vi "Read_File_and_Set_Last_Modified.vi"(5 "file path":path) -> (0 "error out":errorcluster, 1 "string":string, 2 "file path Out":path)   [LabVIEW 2020]
uses:
  Globals/Trav_pos_global.vi
panel:
  out "substring":string
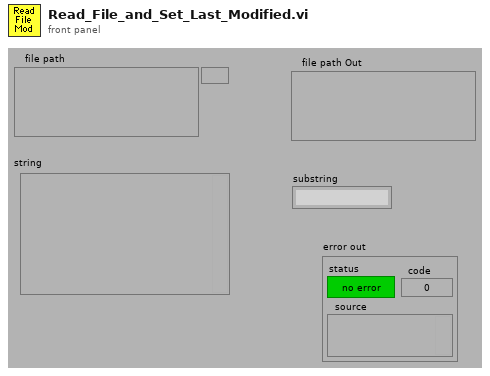
[diagram p1: front panel]
types:
  T1 = enum16{"deny read/write", "deny write-only", "deny none"}
  T2 = enum16{"open", "replace", "create", "open or create", "replace or create", "replace or create with confirmation"}
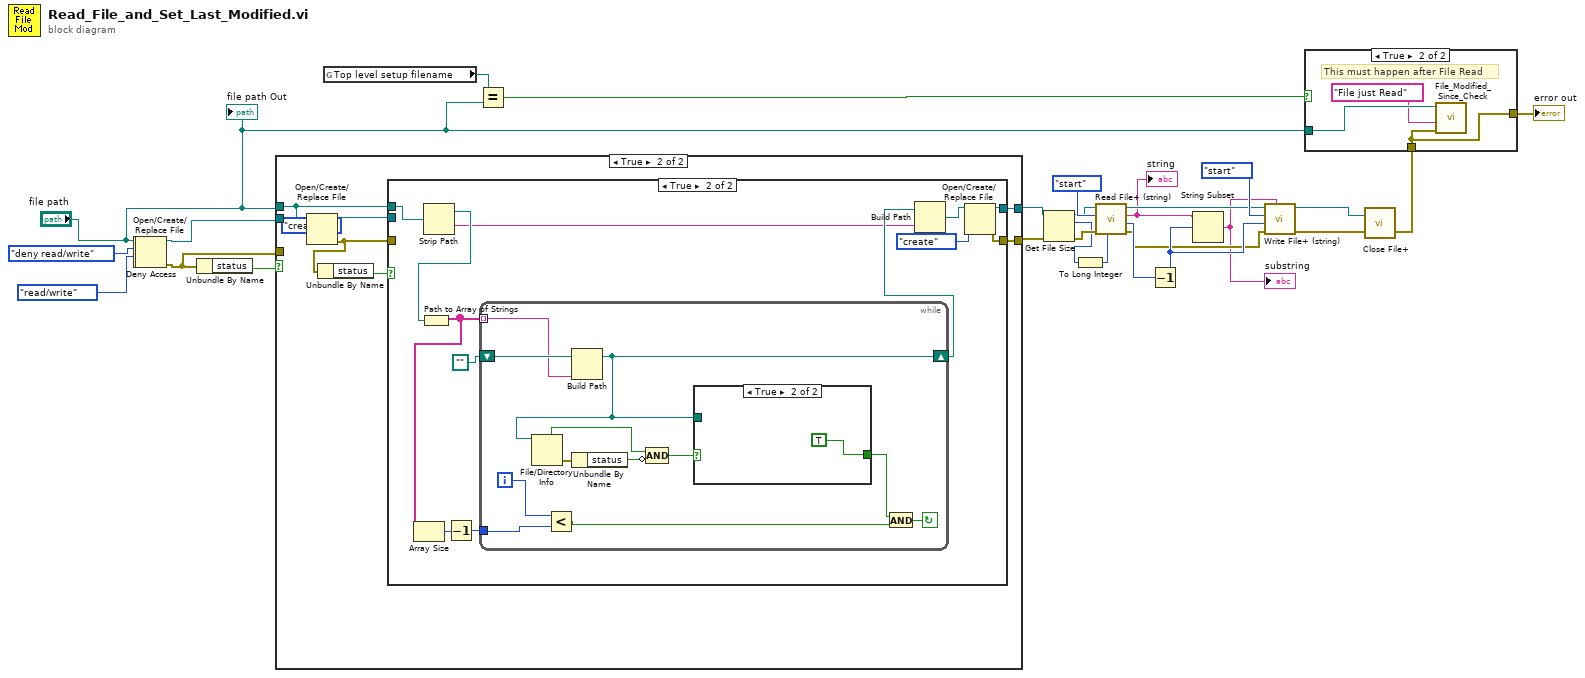
[diagram p0: block diagram]
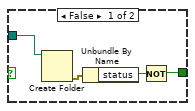
[diagram p5: hidden frame]
diagram:
  n1 = Open/Create/Replace File(file path (use dialog)="file path", access (0:read/write)=enum16{"read/write", "read-only", "write-only"}."read/write") -> (refnum out=w21:refnum<file>, error out=w22:errorcluster)  [unwired: 1 in, 4 out]
  n2 = Deny Access(4:w22, 6:T1."deny read/write" ("deny mode (2)"), 7:w21) -> (0:w23:errorcluster, 3:w26:refnum<file>)
  n3 = Unbundle By Name(w23) -> ("status"=w27:bool)
  n4 = case shown="True" w27 {
    tunnel: "file path" -> [_ w34]
    tunnel: w26 -> [w30 _]
    tunnel: [w30 w37] -> w12
    tunnel: [w29 w36] -> w10
    tunnel: w23 -> [w29 _]
    frame False {
    }
    frame True {
      n5 = Open/Create/Replace File(file path (use dialog)=w34, operation (0:open)=T2."create") -> (refnum out=w33:refnum<file>, error out=w32:errorcluster)  [unwired: 1 in, 4 out]
      n6 = Unbundle By Name(w32) -> ("status"=w35:bool)
      n7 = case shown="True" w35 {
        tunnel: w34 -> [_ w45]
        tunnel: [w39 w48] -> w37
        tunnel: [w38 w47] -> w36
        tunnel: w33 -> [w39 _]
        tunnel: w32 -> [w38 _]
        frame False {
        }
        frame True {
          n8 = Strip Path(path=w45) -> (stripped path=w44:path, name=w42:string)
          n9 = Path to Array of Strings(0:w44) -> (2:w50:string[])  [unwired: 1 out]
          n10 = Array Size(array=w50) -> (size(s)=w51:i32)
          n11 = Decrement(x=w51) -> (x-1=w49:i32)
          n12 = while {
            tunnel: w49 -> [w60]
            shift-left: path "" ("appended path") -> [w63]
            shift-right: [w56] -> w43
            tunnel: w50 -> [w62] mode=indexing
            i -> [w61]
            stop <- w58 continue-if-true
            n13 = Less?(x=w61, y=w60) -> (x < y?=w59:bool)
            n14 = Build Path(base path=w63, name or relative path=w62) -> (appended path=w56:path)
            n15 = File/Directory Info(path=w56) -> (directory=w53:bool, error out=w55:errorcluster)  [unwired: 1 in, 5 out]
            n16 = Unbundle By Name(w55) -> ("status"=w54:bool)
            n17 = Compound Arithmetic op=AND(w53, invert w54) -> (w52:bool)
            n18 = case shown="True" w52 {
              tunnel: w56 -> [w67 _]
              tunnel: [w64 TRUE] -> w57
              frame False {
                n19 = Create Folder(path (use dialog)=w67) -> (error out=w66:errorcluster)  [unwired: 1 in, 3 out]
                n20 = Unbundle By Name(w66) -> ("status"=w65:bool)
                n21 = Not(x=w65) -> (.not. x?=w64:bool)
              }
              frame True {
              }
            }
            n22 = And(x=w57, y=w59) -> (x .and. y?=w58:bool)
          }
          n23 = Build Path(base path=w43, name or relative path=w42) -> (appended path=w41:path)
          n24 = Open/Create/Replace File(file path (use dialog)=w41, operation (0:open)=T2."create") -> (refnum out=w48:refnum<file>, error out=w47:errorcluster)  [unwired: 1 in, 4 out]
        }
      }
    }
  }
  n25 = global read "Trav_pos_global.vi" "Top level setup filename"() -> (w4:path)
  n26 = Equal?(x=w4, y="file path") -> (x = y?=w5:bool)
  n27 = Get File Size(file=w12, error in=w10) -> (refnum out=w11:refnum<file>, size (in bytes)=w8:i64, 0:w9:errorcluster)
  n28 = To Long Integer(number=w8) -> (32bit integer=w7:i32)
  n29 = call <vilib>:"Read File+ (string).vi"("count"=w7, "error in (no error)"=w9, "pos mode (rel. to current:2)"=enum16{"start", "end", "current"}."start", "refnum"=w11) -> ("error out"=w15:errorcluster, "mark after read (bytes)"=w18:i32, "string"=w6:string, "dup refnum"=w14:refnum<file>)  [unwired: 1 in, 3 out]
  "string" <- w6
  n30 = Decrement(x=w18) -> (x-1=w16:i32)
  n31 = String Subset(string=w6, offset (0)=w16) -> (substring=w13:string)  [unwired: 1 in]
  "substring" <- w13
  n32 = call <vilib>:"Write File+ (string).vi"("string"=w13, "error in (no error)"=w15, "pos offset (bytes:0)"=w16, "pos mode (rel. to end:1)"=enum16{"start", "end", "current"}."start", "refnum"=w14) -> ("error out"=w25:errorcluster, "dup refnum"=w24:refnum<file>)  [unwired: 3 out]
  n33 = call <vilib>:"Close File+.vi"("error in (no error)"=w25, "refnum"=w24) -> ("error out"=w1:errorcluster)  [unwired: 5 out]
  n34 = case shown="True" w5 {
    tunnel: "file path" -> [_ w72]
    tunnel: [w69 w70] -> w2
    tunnel: w1 -> [w69 w70]
    frame False {
    }
    frame True {
      # "This must happen after File Read"
      n35 = call "File_Modified_Since_Check.vi"("error in"=w70, "mode"="File just Read", "File Path"=w72) -> ()  [unwired: 5 in, 2 out]
    }
  }
  "error out" <- w2
  "file path Out" <- "file path"
